vi "Utility.FindNewDataFile.vi"(8 "error in (no error)":errorcluster, 9 "LookupTable":variant, 11 "Parameters":T1={"Global.ResultsPath"=path "C:/Conti/Logs", "Global.TempPath"=path "C:/Conti/Temp", "Global.RemotePath"=path "d:/Conti/Logs", "TDMS.AnalysisVIs"=[], "TDMS.ReportPassed?"=FALSE, "TDMS.GroupChannels?"=FALSE}) -> (0 "error out":errorcluster, 1 "LookupTable out":variant, 2 "Found":bool, 3 "Data Path":path)   [LabVIEW 2015, in "Analysis.lvlib"]
uses:
  Analysis.lvlib
  Types/Analysis.GUI.Parameters.ctl
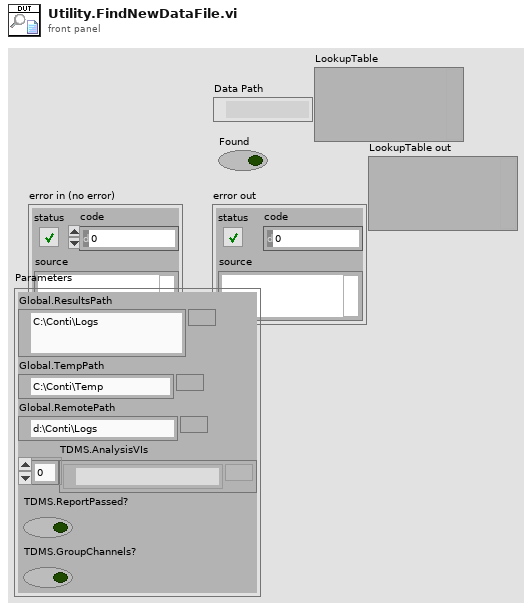
[diagram p1: front panel]
types:
  T1 = typedef "Analysis.lvlib/Analysis.GUI.Parameters.ctl" = cluster{"Global.ResultsPath":path, "Global.TempPath":path, "Global.RemotePath":path, "TDMS.AnalysisVIs":path[], "TDMS.ReportPassed?":bool, "TDMS.GroupChannels?":bool}
  T2 = cluster{"size":i64, "millisecond timer value":u32}
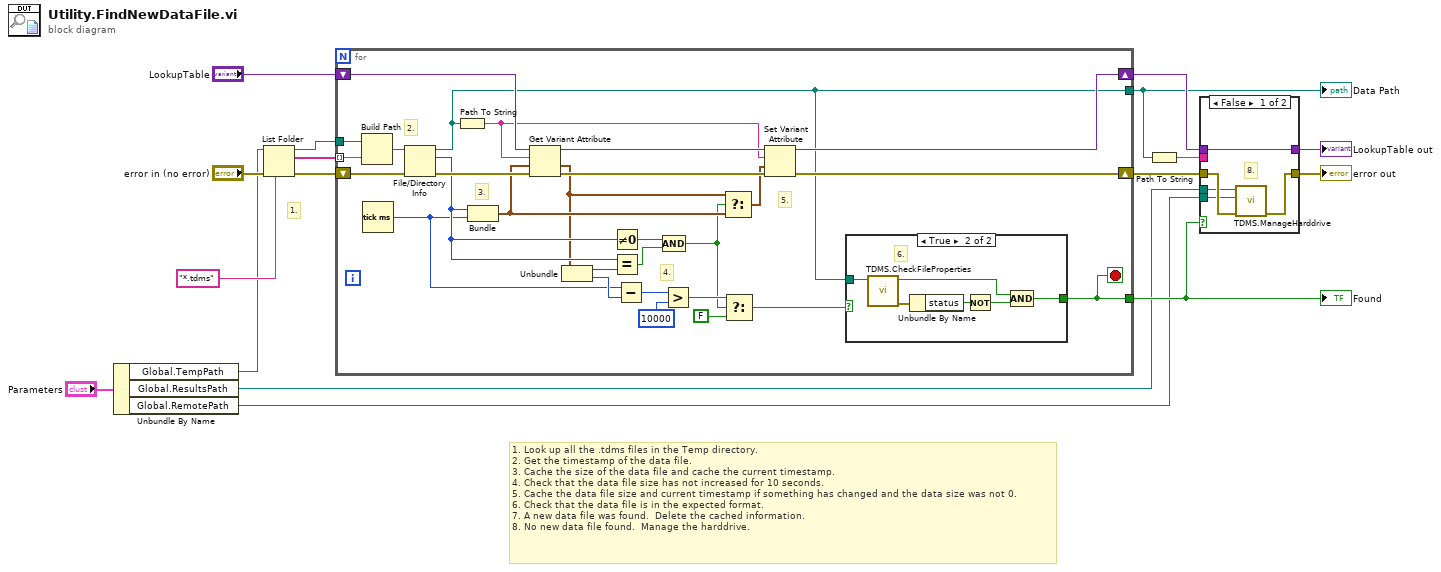
[diagram p0: block diagram]
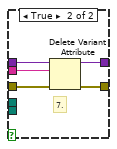
[diagram p3: hidden frame]
diagram:
  # "1. Look up all the .tdms files in the Temp directory.\n2. Get the timestamp of the data file.\n3. Cache the size of the data file and cache the current timestamp.\n4. Check that the data file size has not increased for 10 seconds.\n5. Cache the data file size and current timestamp if something has changed and the data size was not 0.\n6. Check that the data file is in the expected format.\n7. A new data file was found.  Delete the cached information.\n8. No new data file found.  Manage the harddrive."
  # "1."
  n1 = Unbundle By Name("Parameters") -> ("Global.TempPath"=w1:path, "Global.ResultsPath"=w3:path, "Global.RemotePath"=w2:path)
  n2 = List Folder(path=w1, pattern="*.tdms", error in="error in (no error)") -> (path out=w13:path, filenames=w14:string[], error out=w15:errorcluster)  [unwired: 1 in, 1 out]
  n3 = for {
    tunnel: w13 -> [w45]
    tunnel: w14 -> [w44] mode=indexing
    shift-right: [w37] -> w11
    shift-left: w15 -> [w43]
    tunnel: [w32] -> w5
    tunnel: [w34] -> w6
    shift-right: [w35] -> w9
    shift-left: "LookupTable" -> [w40]
    stop <- w32 stop-if-true
    # "5."
    # "4."
    # "3."
    # "2."
    n4 = Build Path(base path=w45, name or relative path=w44) -> (appended path=w42:path)
    n5 = Tick Count (ms)() -> (millisecond timer value=w23:u32)
    n6 = File/Directory Info(path=w42, error in=w43) -> (path out=w34:path, size=w27:i64, error out=w41:errorcluster)  [unwired: 4 out]
    n7 = Path To String(path=w34) -> (string=w36:string)
    n8 = Bundle("size"=w27, "millisecond timer value"=w23) -> (w28:T2)  [unwired: 1 in]
    n9 = Get Variant Attribute(Variant=w40, name=w36, default value (empty Variant)=w28, error in=w41) -> (duplicate Variant=w39:variant, value=w25:T2, error out=w38:errorcluster)  [unwired: 1 out]
    n10 = Unbundle(w25) -> ("size"=w29:i64, "millisecond timer value"=w24:u32)
    n11 = Not Equal To 0?(x=w27) -> (x != 0?=w31:bool)
    n12 = Equal?(x=w27, y=w29) -> (x = y?=w30:bool)
    n13 = Subtract(x=w23, y=w24) -> (x-y=w21:u32)
    n14 = Compound Arithmetic op=AND(w31, w30) -> (w18:bool)
    n15 = Greater?(x=w21, y=u32 10000) -> (0:w19:bool)
    n16 = Select(t=w25, s=w18, f=w28) -> (s? t:f=w26:T2)
    n17 = Select(t=w19, s=w18, f=FALSE) -> (s? t:f=w33:bool)
    n18 = Set Variant Attribute(Variant=w39, name=w36, value=w26, error in=w38) -> (Variant out=w35:variant, error out=w37:errorcluster)  [unwired: 1 out]
    n19 = case shown="True" w33 {
      selector: w33 -> [w46 _]
      tunnel: w34 -> [_ w50]
      tunnel: [w46 w48] -> w32
      frame False {
      }
      frame True {
        # "6."
        n20 = call "TDMS.CheckFileProperties.vi"("Data"=w50) -> ("error out"=w49:errorcluster, "Found All"=w47:bool)  [unwired: 9 in]
        n21 = Unbundle By Name(w49) -> ("status"=w52:bool)
        n22 = Not(x=w52) -> (.not. x?=w51:bool)
        n23 = Compound Arithmetic op=AND(w47, w51) -> (w48:bool)
      }
    }
  }
  "Data Path" <- w6
  "Found" <- w5
  n24 = Path To String(path=w6) -> (string=w7:string)
  n25 = case shown="False" w5 {
    tunnel: w11 -> [w56 w62]
    tunnel: [w55 w61] -> w10
    tunnel: w9 -> [w57 w60]
    tunnel: [w57 w59] -> w8
    tunnel: w7 -> [_ w58]
    tunnel: w3 -> [w54 _]
    tunnel: w2 -> [w53 _]
    frame False {
      # "8."
      n26 = call "TDMS.ManageHarddrive.vi"("error in"=w56, "Remote Path"=w53, "Results Path"=w54) -> ("error out"=w55:errorcluster)  [unwired: 8 in]
    }
    frame True {
      # "7."
      n27 = Delete Variant Attribute(4:w62, 6:w58, 7:w60) -> (0:w61:errorcluster, 3:w59:variant)  [unwired: 1 out]
    }
  }
  "error out" <- w10
  "LookupTable out" <- w8
